vi "Epoxy Actuate Valves.vi"(8 "error in (no error)":errorcluster, 10 "Valves Control":T1, 11 "VISA Refnum in":refnum<visa-resource-name>) -> (0 "error out":errorcluster, 3 "String":string)   [LabVIEW 2020]
uses:
  controls/Valves Radio.ctl
  <instrlib>/Agilent 34970/Agilent 34970.lvlib
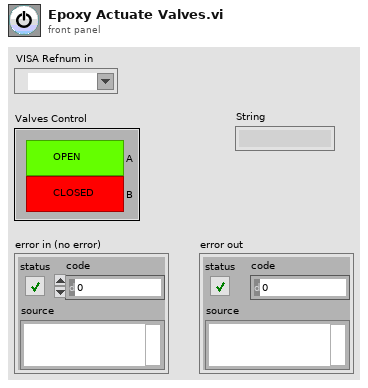
[diagram p1: front panel]
types:
  T1 = typedef "Valves Radio.ctl" = enum32{"A", "B"}
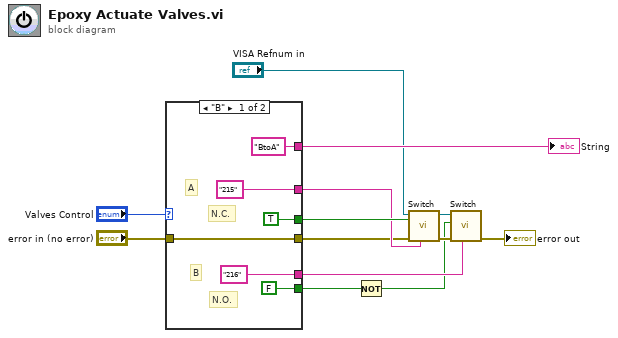
[diagram p0: block diagram]
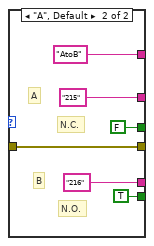
[diagram p2: hidden frame]
diagram:
  n1 = case shown="\"B\"" "Valves Control" {
    tunnel: "error in (no error)" -> [w19 w25]
    tunnel: [w19 w25] -> w4
    tunnel: ["215" "215"] -> w7
    tunnel: ["216" "216"] -> w8
    tunnel: [FALSE ("Open/Close (F:Close)") TRUE ("Open/Close (F:Close)")] -> w10
    tunnel: [TRUE ("Open/Close (F:Close)") FALSE ("Set/Check (F:Set)")] -> w9
    tunnel: ["BtoA" "AtoB"] -> w11
    frame "B" {
      # "N.O."
      # "N.C."
      # "B"
      # "A"
    }
    frame "A", Default {
      # "N.O."
      # "N.C."
      # "B"
      # "A"
    }
  }
  "String" <- w11
  n2 = Not(x=w10) -> (.not. x?=w1:bool)
  n3 = call <instrlib>:"Switch.vi"("Channel List(empty)"=w7, "error in (no error)"=w4, "Open/Close (F:Close)"=w9, "VISA Resource Name"="VISA Refnum in") -> ("error out"=w5:errorcluster, "VISA Resource Name Out"=w6:refnum<visa-resource-name>)  [unwired: 5 in, 1 out]
  n4 = call <instrlib>:"Switch.vi"("Channel List(empty)"=w8, "error in (no error)"=w5, "Open/Close (F:Close)"=w1, "VISA Resource Name"=w6) -> ("error out"=→"error out":errorcluster)  [unwired: 5 in, 2 out]
